vi "PH_Beckhoff_PP_PU.set i Attr and start DIM Services for RR.vi"(3 "error in":errorcluster, 4 "Values":T4, 5 "PU Type":T3=enum."PA 19mm") -> (0 "error out":errorcluster, 1 "RossRelais":T2(array[cluster]) {"Status"."Status" items=["no info", "off/false/out", "on/true/in", "Failure", "Alarm", "Status 1", "Status 2", "Status 3"]})   [LabVIEW 2014, in "PH_Beckhoff_PP_PU.lvlib"]
uses:
  PH_Beckhoff_PP_PU.lvlib
  PH_Beckhoff/PH_Beckhoff.Values.ctl
  PH_Beckhoff/PH_Beckhoff.Sonderklemmen Inputs.ctl
  PH_Beckhoff/PH_Beckhoff.Analog Inputs.ctl
  PH_Beckhoff/PH_Beckhoff.Scaling Type.ctl
  PH_Beckhoff/PH_Beckhoff.Analog Outputs.ctl
  PH_Beckhoff/PH_Beckhoff.Digital Inputs.ctl
  PH_Beckhoff/PH_Beckhoff.Digital Outputs.ctl
  PH_Beckhoff_PP_PU.PU Rack Type.ctl
  PH_Basics/PH_StatusHandler/PH_StatusHandler.Status.ctl
  PH_Beckhoff_PP_PU.RR Tags.ctl
  CSlibraries-extern/DimLVEvent/LVDimInterface/LVDimInterface.lvlib
  PH_Basics/PH_StatusHandler/PH_StatusHandler.lvlib
  PH_Beckhoff/PH_Beckhoff.lvlib
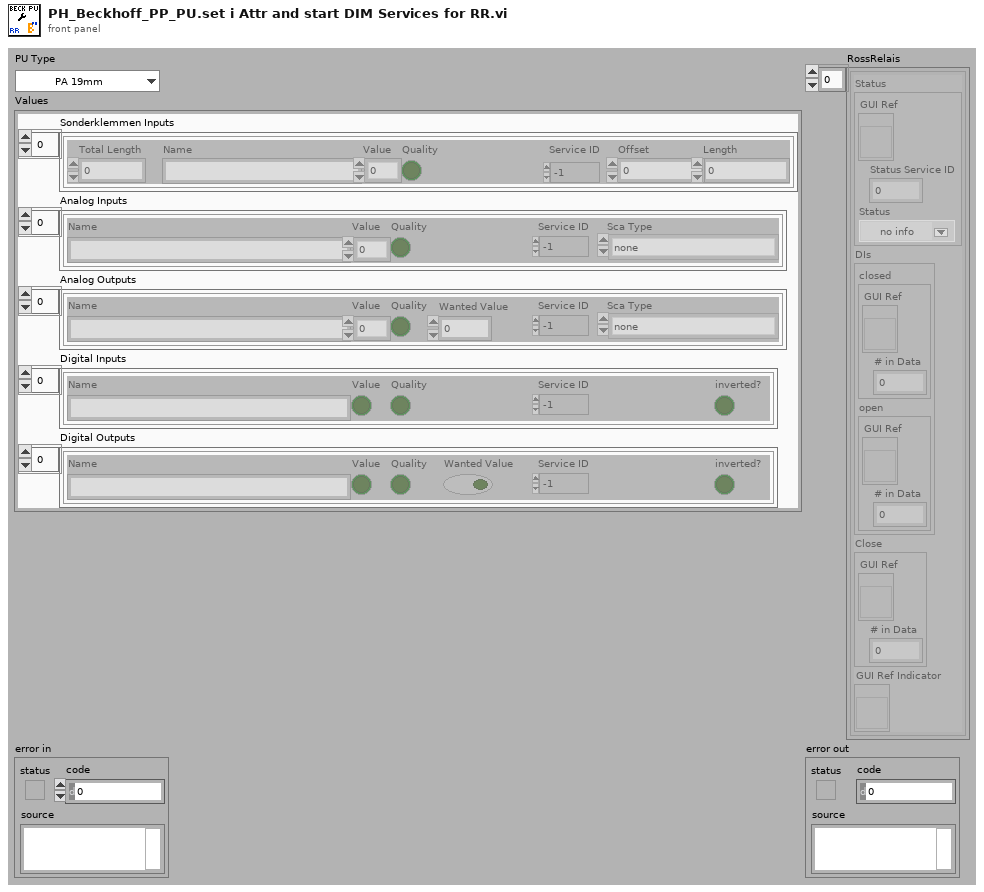
[diagram p1: front panel]
types:
  T1 = typedef "PH_StatusHandler.lvlib/PH_StatusHandler.Status.ctl" = i16
  T2 = cluster{"Status":cluster{"GUI Ref":refnum<vi>, "Status Service ID":i32, "Status":T1}, "DIs":cluster{"closed":cluster{"GUI Ref":refnum<vi>, "# in Data":i32}, "open":cluster{"GUI Ref":refnum<vi>, "# in Data":i32}}, "Close":cluster{"GUI Ref":refnum<vi>, "# in Data":i32}, "GUI Ref Indicator":refnum<vi>}[]
  T3 = typedef "PH_Beckhoff_PP_PU.lvlib/PH_Beckhoff_PP_PU.PU Rack Type.ctl" = enum16{"no Info", "PA 19mm", "PA 45mm", "MA PU 1 and 2", "MA PU 3 and 4", "MA PU 5 and 6", "MA FR and PILC"}
  T4 = typedef "PH_Beckhoff.lvlib/PH_Beckhoff.Values.ctl" = cluster{"Sonderklemmen Inputs":T5, "Analog Inputs":T6, "Analog Outputs":T8, "Digital Inputs":T9, "Digital Outputs":T10}
  T5 = typedef "PH_Beckhoff.lvlib/PH_Beckhoff.Sonderklemmen Inputs.ctl" = cluster{"Total Length":u32, "Name":string, "Value":u64, "Quality":bool, "Service ID":i32, "Offset":u32, "Length":u32}[]
  T6 = typedef "PH_Beckhoff.lvlib/PH_Beckhoff.Analog Inputs.ctl" = cluster{"Name":string, "Value":u32, "Quality":bool, "Service ID":i32, "Sca Type":T7}[]
  T7 = typedef "PH_Beckhoff.lvlib/PH_Beckhoff.Scaling Type.ctl" = enum16{"none", "0 ... 15 Bit -> 0 ... 5", "0 ... 15 Bit -> 0 ... 10", "0 ... 15 Bit -> 0 ... 25", "0 ... 15 Bit -> 4 ... 20", "0 ... 15 Bit -> 0 ... 1", "0 ... 15 Bit -> 0 ... 20000", "0 ... 15 Bit -> 0 ... 24000"}
  T8 = typedef "PH_Beckhoff.lvlib/PH_Beckhoff.Analog Outputs.ctl" = cluster{"Name":string, "Value":u32, "Quality":bool, "Wanted Value":u32, "Service ID":i32, "Sca Type":T7}[]
  T9 = typedef "PH_Beckhoff.lvlib/PH_Beckhoff.Digital Inputs.ctl" = cluster{"Name":string, "Value":bool, "Quality":bool, "Service ID":i32, "inverted?":bool}[]
  T10 = typedef "PH_Beckhoff.lvlib/PH_Beckhoff.Digital Outputs.ctl" = cluster{"Name":string, "Value":bool, "Quality":bool, "Wanted Value":bool, "Service ID":i32, "inverted?":bool}[]
  T11 = typedef "PH_Beckhoff_PP_PU.lvlib/PH_Beckhoff_PP_PU.RR Tags.ctl" = enum16{"open", "closed", "close", "Status"}
  T12 = typedef "PH_PP_Common.lvlib/PH_PP_Common.PUs.ctl" = enum16{"no Info", "PA-19mm-1", "PA-19mm-2", "PA-45mm-PILC", "PA-45mm-MAIN", "MA-PU-1", "MA-PU-2", "MA-PU-3", "MA-PU-4", "MA-PU-5", "MA-PU-6", "MA-FR", "MA-PILC", "PA-45mm-DP"}
  T13 = cluster{"Status":cluster{"GUI Ref":refnum<vi>, "Status Service ID":i32, "Status":T1}, "DIs":cluster{"closed":cluster{"GUI Ref":refnum<vi>, "# in Data":i32}, "open":cluster{"GUI Ref":refnum<vi>, "# in Data":i32}}, "Close":cluster{"GUI Ref":refnum<vi>, "# in Data":i32}, "GUI Ref Indicator":refnum<vi>}
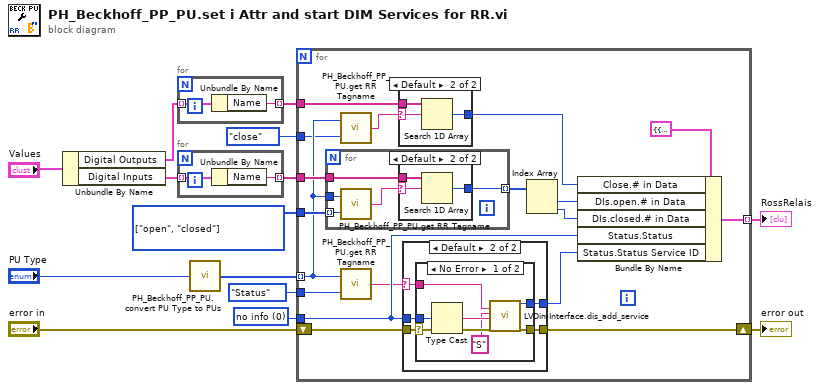
[diagram p0: block diagram]
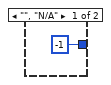
[diagram p2: hidden frame]
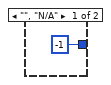
[diagram p3: hidden frame]
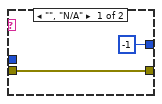
[diagram p4: hidden frame]
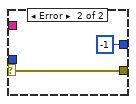
[diagram p5: hidden frame]
diagram:
  w8 = T11[] [enum."open", enum."closed"] items=["open", "closed", "close", "Status"]
  w10 = T1 0 items=["no info", "off/false/out", "on/true/in", "Failure", "Alarm", "Status 1", "Status 2", "Status 3"] ("Status")
  n1 = Unbundle By Name("Values") -> ("Digital Outputs"=w5:T10, "Digital Inputs"=w7:T9)
  n2 = for {
    tunnel: w5 -> [w16] mode=indexing
    tunnel: [w15] -> w4 mode=indexing
    n3 = Unbundle By Name(w16) -> ("Name"=w15:string)
  }
  n4 = for {
    tunnel: w7 -> [w18] mode=indexing
    tunnel: [w17] -> w6 mode=indexing
    n5 = Unbundle By Name(w18) -> ("Name"=w17:string)
  }
  n6 = call "PH_Beckhoff_PP_PU.convert PU Type to PUs.vi"("PU Type"="PU Type") -> ("PUs"=w11:T12[])
  n7 = for {
    shift-right: [w35] -> w14
    shift-left: "error in" -> [w36]
    tunnel: [w31] -> w1 mode=indexing
    tunnel: w11 -> [w24] mode=indexing
    tunnel: PH_Beckhoff_PP_PU.RR_Tags."Status" ("Ross Relais Tag") -> [w32]
    tunnel: w10 -> [w34]
    tunnel: w8 -> [w29]
    tunnel: w6 -> [w25]
    tunnel: w4 -> [w21]
    tunnel: PH_Beckhoff_PP_PU.RR_Tags."close" ("Ross Relais Tag") -> [w20]
    n8 = for {
      tunnel: w24 -> [w45]
      tunnel: w29 -> [w44] mode=indexing
      tunnel: [w43] -> w28 mode=indexing
      tunnel: w25 -> [w41]
      n9 = call "PH_Beckhoff_PP_PU.get RR Tagname.vi"("Ross Relais Tag"=w44, "PU"=w45) -> ("RR Tagname"=w42:string)
      n10 = case shown="Default" w42 {
        selector: w42 -> [_ w48]
        tunnel: [-1 ("index of element") w49] -> w43
        tunnel: w41 -> [_ w47]
        frame "", "N/A" {
        }
        frame Default {
          n11 = Search 1D Array(1D array=w47, element=w48) -> (index of element=w49:i32)  [unwired: 1 in]
        }
      }
    }
    n12 = call "PH_Beckhoff_PP_PU.get RR Tagname.vi"("Ross Relais Tag"=w20, "PU"=w24) -> ("RR Tagname"=w23:string)
    n13 = call "PH_Beckhoff_PP_PU.get RR Tagname.vi"("Ross Relais Tag"=w32, "PU"=w24) -> ("RR Tagname"=w33:string)
    n14 = case shown="Default" w23 {
      selector: w23 -> [_ w39]
      tunnel: [-1 ("index of element") w40] -> w22
      tunnel: w21 -> [_ w38]
      frame "", "N/A" {
      }
      frame Default {
        n15 = Search 1D Array(1D array=w38, element=w39) -> (index of element=w40:i32)  [unwired: 1 in]
      }
    }
    n16 = case shown="Default" w33 {
      selector: w33 -> [_ w52]
      tunnel: w36 -> [w51 w56]
      tunnel: [w51 w55] -> w35
      tunnel: [-1 ("my_serviceID") w54] -> w30
      tunnel: w34 -> [_ w53]
      frame "", "N/A" {
      }
      frame Default {
        n17 = case shown="No Error" w56 {
          selector: w56 -> [w61 w65]
          tunnel: [w63 -1 ("my_serviceID")] -> w54
          tunnel: [w62 w65] -> w55
          tunnel: w53 -> [w60 _]
          tunnel: w52 -> [w57 _]
          frame No Error {
            n18 = Type Cast(x=w60) -> (*(type *) &x=w59:string)  [unwired: 1 in]
            n19 = call "LVDimInterface.dis_add_service.vi"("serviceName"=w57, "typeDescriptor"="S", "data"=w59, "error in (no error)"=w61) -> ("my_serviceID"=w63:i32, "error out"=w62:errorcluster)  [unwired: 14 in]
          }
          frame Error {
          }
        }
      }
    }
    n20 = Index Array(array=w28) -> (element #1=w27:i32, element #2=w26:i32)  [unwired: 2 in]
    n21 = Bundle By Name(cluster=T13 {"Status"={"GUI Ref"=refnum, "Status Service ID"=0, "Status"=0}, "DIs"={"closed"={"GUI Ref"=refnum, "# in Data"=0}, "open"={"GUI Ref"=refnum, "# in Data"=0}}, "Close"={"GUI Ref"=refnum, "# in Data"=0}, "GUI Ref Indicator"=refnum} ("RR Data"), "Close.# in Data"=w22, "DIs.open.# in Data"=w27, "DIs.closed.# in Data"=w26, "Status.Status"=w34, "Status.Status Service ID"=w30) -> (w31:T13)
  }
  "error out" <- w14
  "RossRelais" <- w1
